vi "digits_per_micron.vi"(1 "Ch1Range":i32) -> (0 "digital_per_micron":dbl)   [LabVIEW 2018]
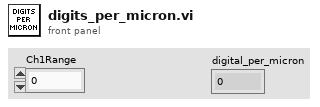
[diagram p1: front panel]
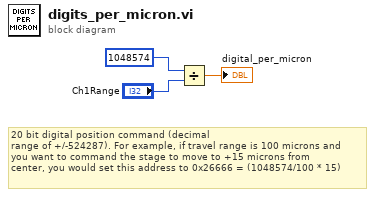
[diagram p0: block diagram]
diagram:
  # "20 bit digital position command (decimal\nrange of +/-524287). For example, if travel range is 100 microns and\nyou want to command the stage to move to +15 microns from\ncenter, you would set this address to 0x26666 = (1048574/100 * 15)"
  n1 = Divide(x=1048574, y="Ch1Range") -> (x/y=→"digital_per_micron":dbl)
